vi "VNA-FMR_out-of-plane.vi"() -> ()   [LabVIEW 2015]
panel:
  out "Email Errors":string
  in  "File Comment":string
  in  "IF Bandwidth":string="10"
  in  "Stop":bool
  out "Status":string
  in  "Field Points":i32=1
  out "Current Set Point":dbl
  out "Current Output":dbl
  in  "Global Finished Email":bool
  in  "Save Directory":path=path "C:/Users/probe_station/Desktop/VNA-FMR_Data"
  in  "Scan Email":bool
  in  "Send File":bool
  out "Frequency":string
  out "Sweep Number":dbl
  out "Average IMAG":cluster{dbl[], dbl[]}(graph)
  out "Average REAL":cluster{dbl[], dbl[]}(graph)
  in  "Field Sweeps":i32=5
  out "Sweep IMAG":cluster{dbl[], dbl[]}(graph)
  out "Sweep REAL":cluster{dbl[], dbl[]}(graph)
  out "VNA IMAG":dbl
  out "Field (Oe)":dbl
  out "VNA REAL":dbl
  in  "FW Bell?":bool
  in  "Response Cal":bool=TRUE
  in  "Port Power Level":string="0"
  in  "Marker Sweep/Time Point":string="3ms"
  in  "VNA CW Sweep Time":string="min"
  in  "VNA number of Points":string="2"
  in  "Power Supply Address":string="1"
  in  "Current Start (A)":dbl
  in  "Current Stop (A)":dbl=70.0
  in  "VNA Address":string="15"
  in  "GaussMeter Address":string="12"
  in  "Start (GHz)":dbl=8.0
  in  "Stop (GHz)":dbl=9.0
  in  "Frequency Points":i32=2
  in  "Recipient's Email Address Address":string
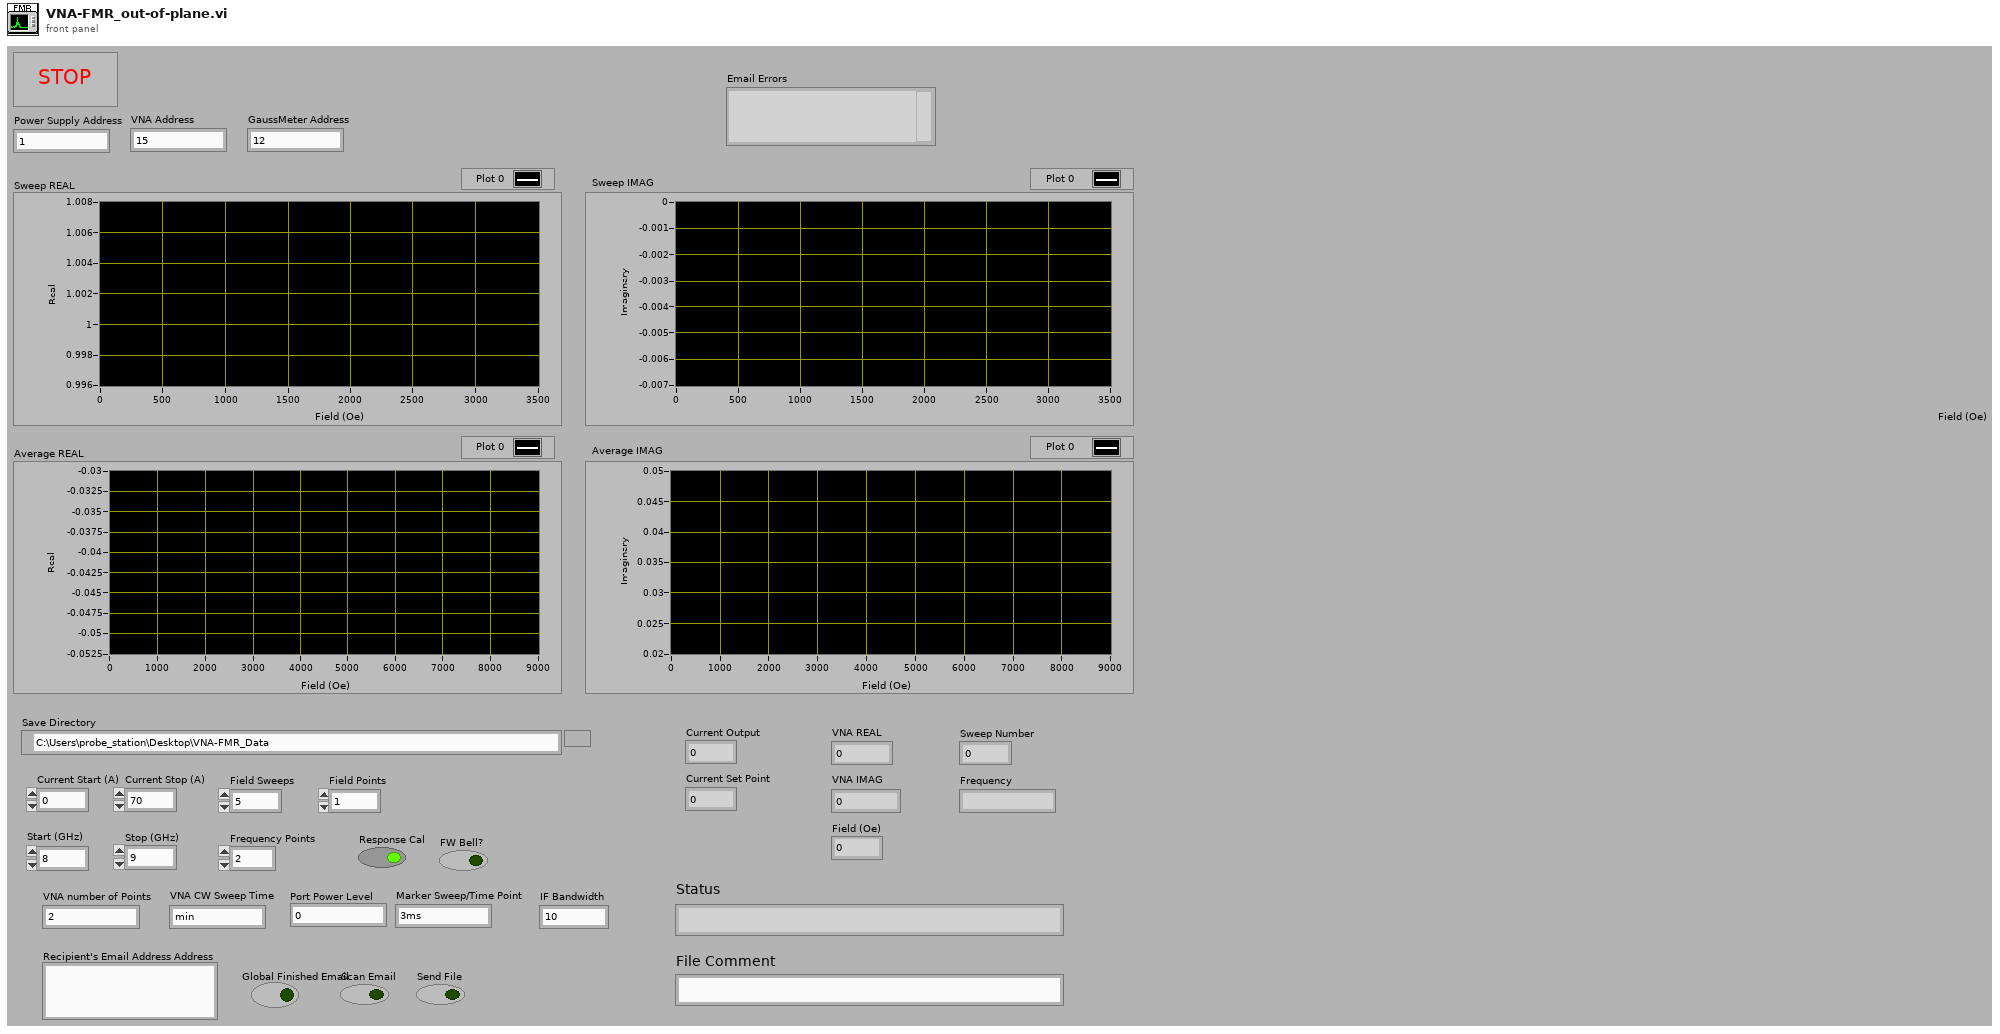
[diagram p1: front panel]
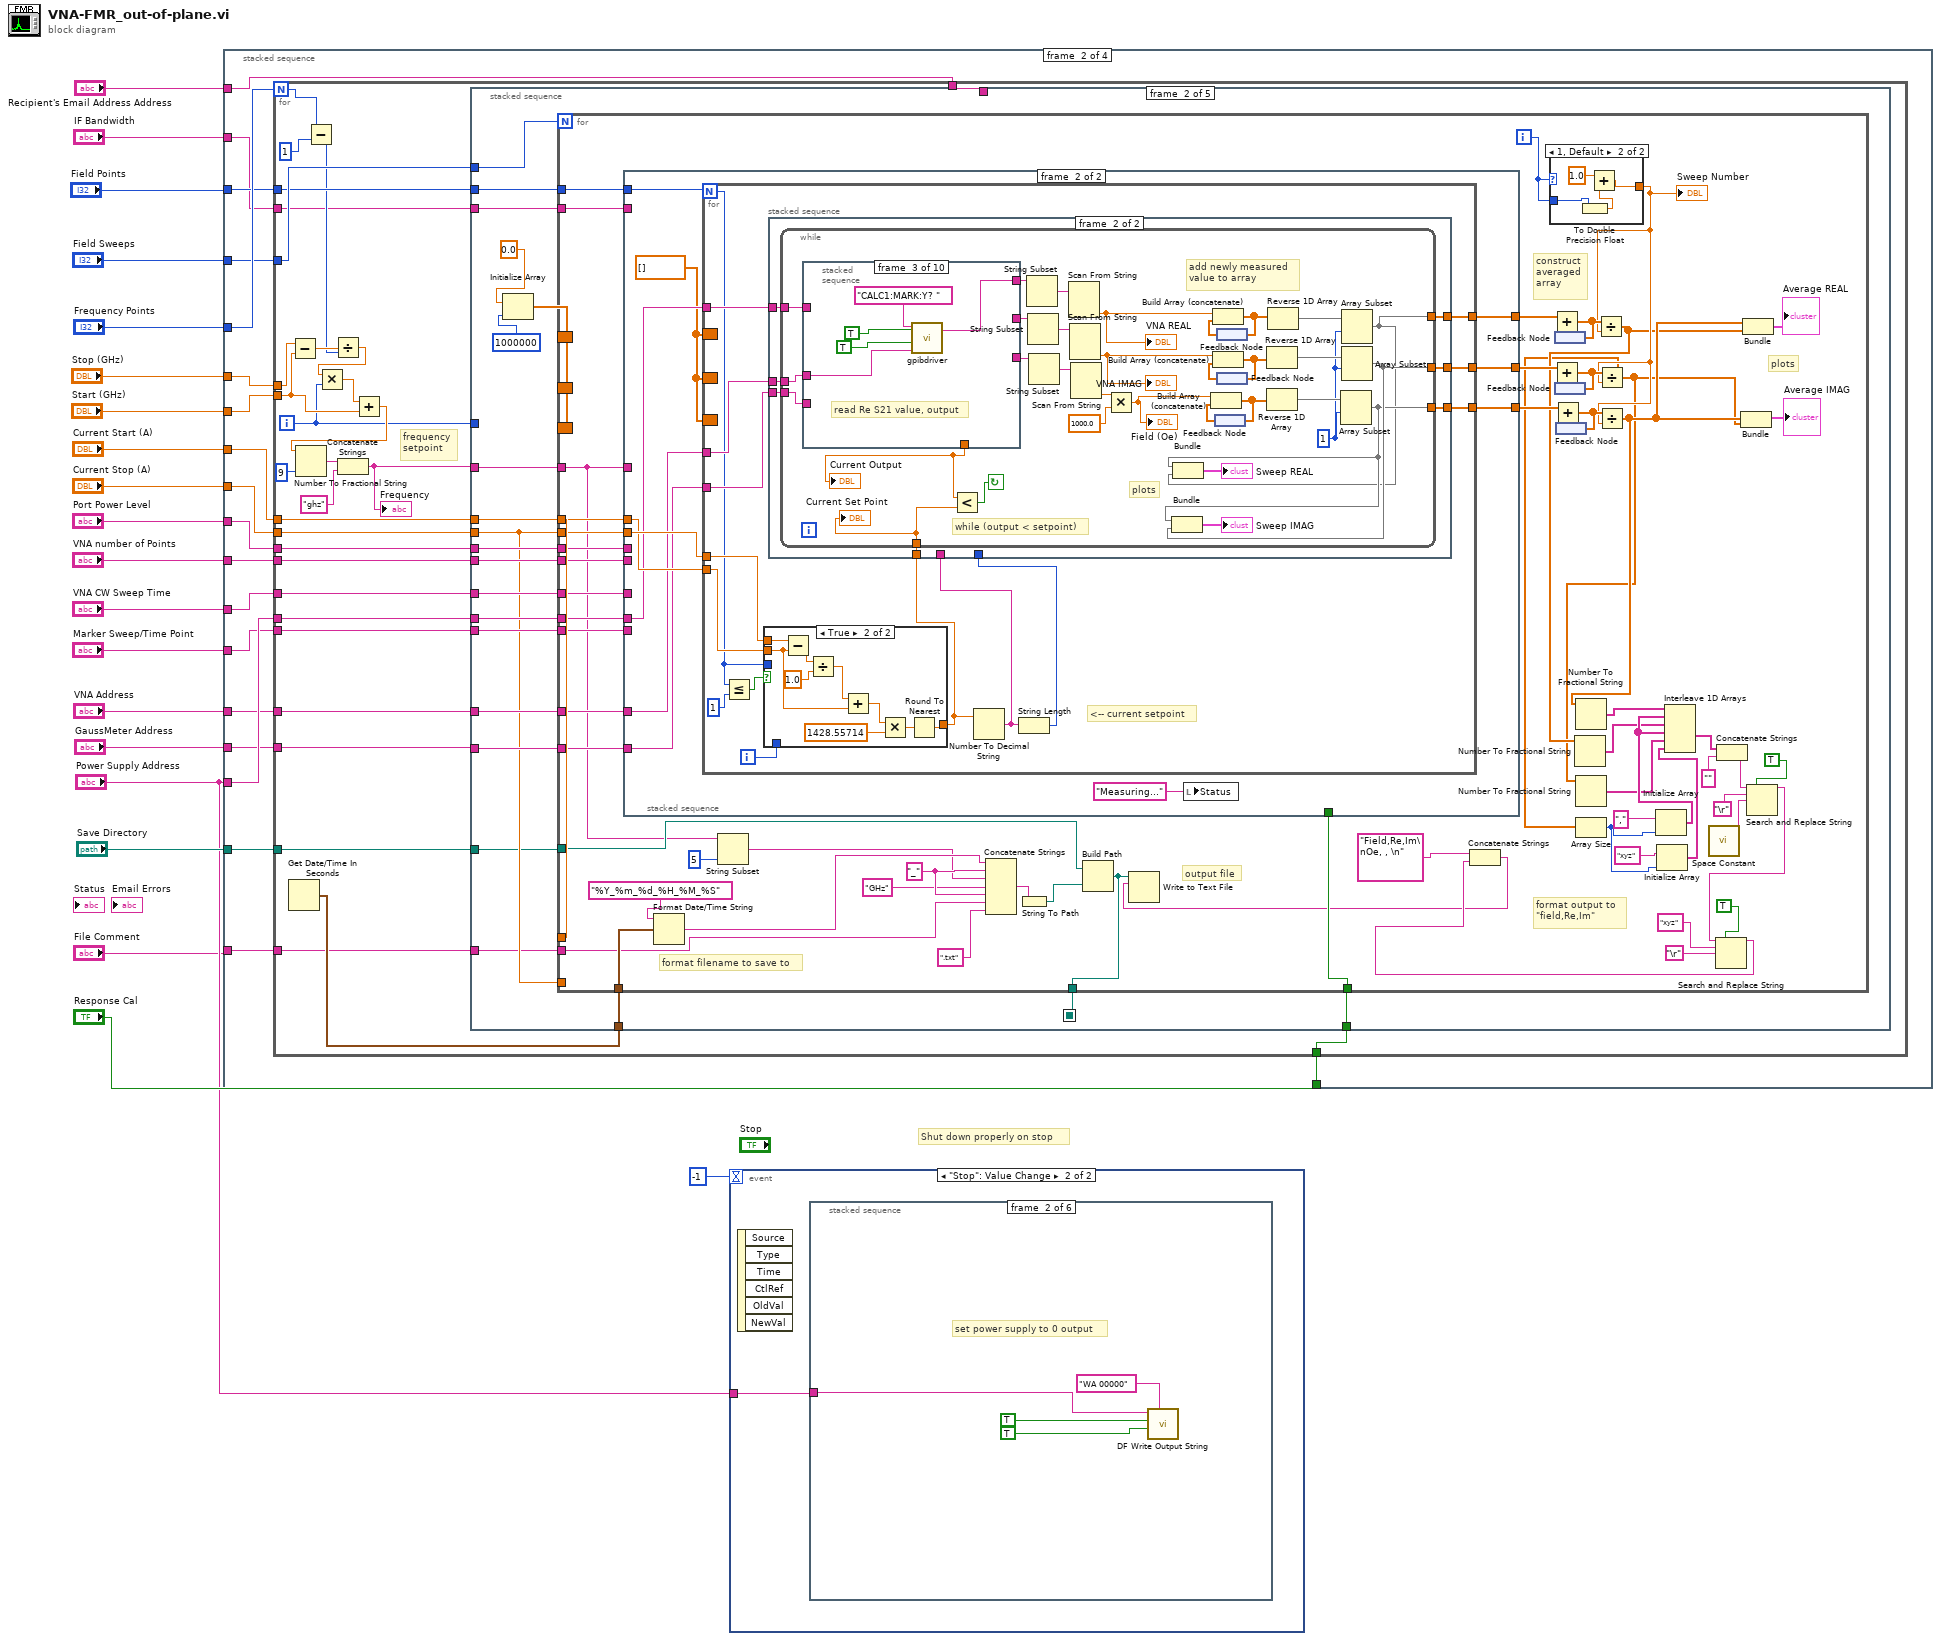
[diagram p0: block diagram]
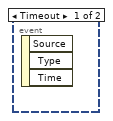
[diagram p2: hidden frame]
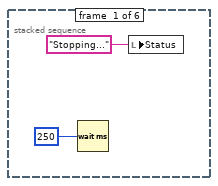
[diagram p3: hidden frame]
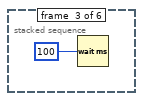
[diagram p4: hidden frame]
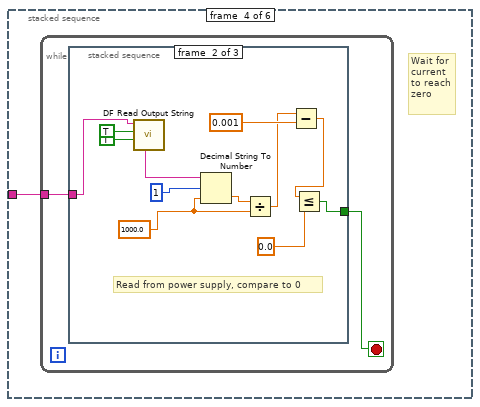
[diagram p5: hidden frame]
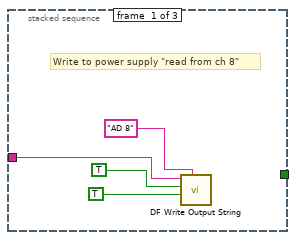
[diagram p6: hidden frame]
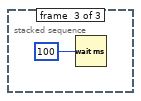
[diagram p7: hidden frame]
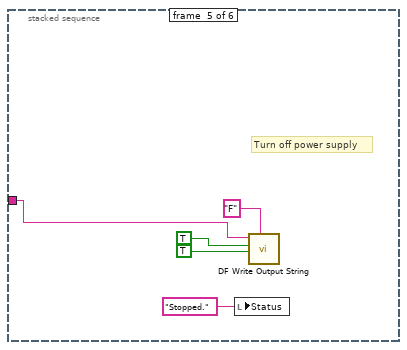
[diagram p8: hidden frame]
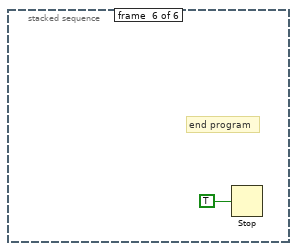
[diagram p9: hidden frame]
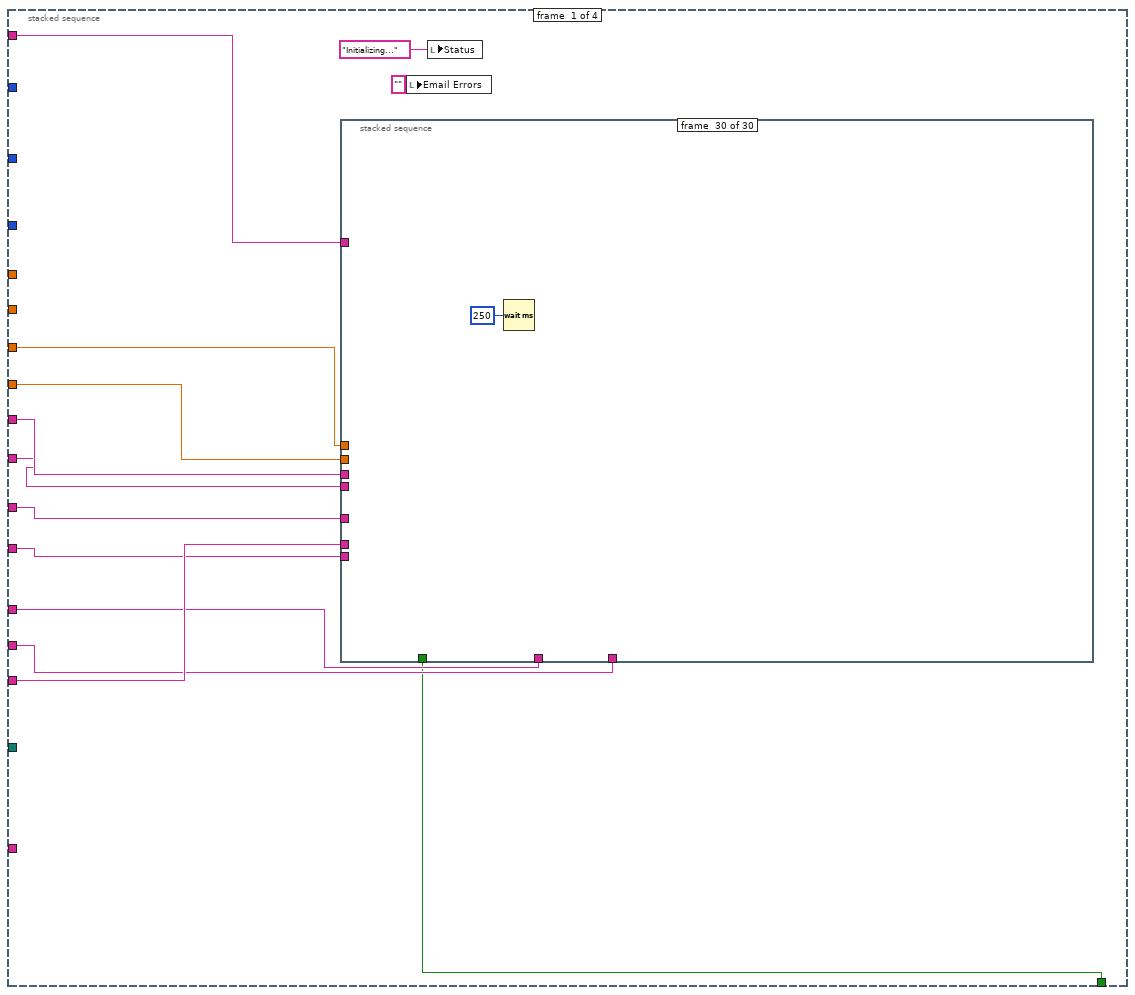
[diagram p10: hidden frame]
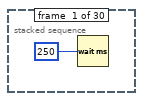
[diagram p11: hidden frame]
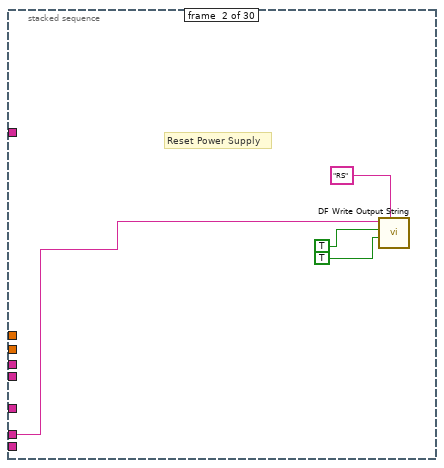
[diagram p12: hidden frame]
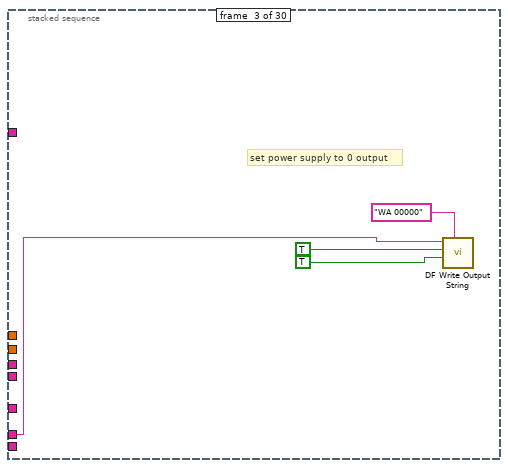
[diagram p13: hidden frame]
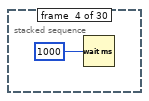
[diagram p14: hidden frame]
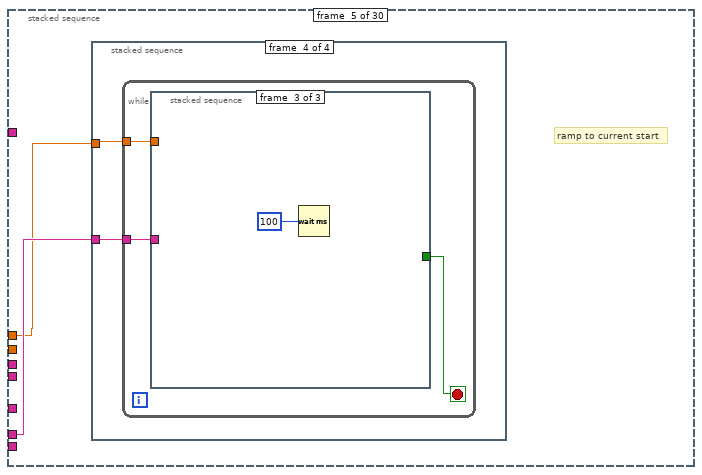
[diagram p15: hidden frame]
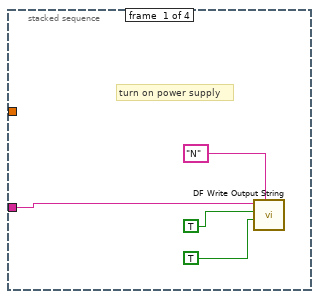
[diagram p16: hidden frame]
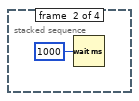
[diagram p17: hidden frame]
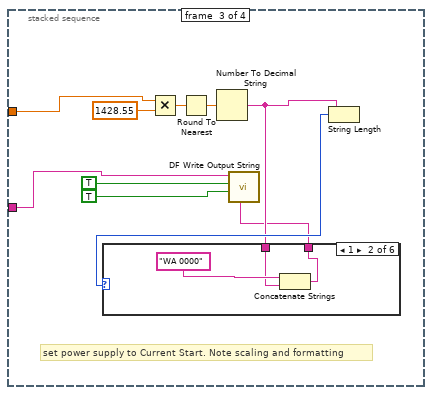
[diagram p18: hidden frame]
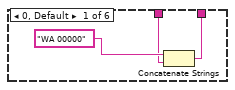
[diagram p19: hidden frame]
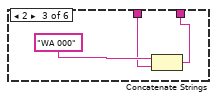
[diagram p20: hidden frame]
diagram:
  # "Shut down properly on stop"
  n1 = stacked-sequence {
    tunnel: "Recipient's Email Address Address" -> [_ w243 w824 _]
    tunnel: "Frequency Points" -> [_ w258 _ _]
    tunnel: "Stop (GHz)" -> [_ w257 _ _]
    tunnel: "Start (GHz)" -> [_ w256 _ _]
    tunnel: "Current Start (A)" -> [w33 w254 _ _]
    tunnel: "Current Stop (A)" -> [w32 w253 _ _]
    tunnel: "Port Power Level" -> [w31 w250 _ _]
    tunnel: "VNA number of Points" -> [w30 w251 _ _]
    tunnel: "VNA CW Sweep Time" -> [w29 w249 _ _]
    tunnel: "Marker Sweep/Time Point" -> [w27 w247 _ _]
    tunnel: "VNA Address" -> [w26 w252 _ _]
    tunnel: "Power Supply Address" -> [w28 w255 w823 _]
    tunnel: "GaussMeter Address" -> [w25 w246 _ _]
    tunnel: "Response Cal" -> [w24 w248 _ _]
    tunnel: "Field Points" -> [_ w245 _ _]
    tunnel: "Field Sweeps" -> [_ w244 _ _]
    tunnel: "Save Directory" -> [_ w242 _ _]
    tunnel: "IF Bandwidth" -> [w22 w241 _ _]
    tunnel: "File Comment" -> [_ w240 w821 _]
    frame #0 {
      n2 = stacked-sequence {
        tunnel: w28 -> [_ w38 w39 _ w45 _ _ _ _ _ _ _ _ _ _ _ _ _ _ _ _ _ _ _ _ _ _ _ _ _]
        tunnel: w33 -> [_ _ _ _ w44 _ _ _ _ _ _ _ _ _ _ _ _ _ _ _ _ _ _ _ _ _ _ _ _ _]
        tunnel: w32 -> [_ _ _ _ _ _ _ _ _ _ _ _ _ _ _ _ _ _ _ _ _ _ _ _ _ _ _ _ _ _]
        tunnel: w26 -> [_ _ _ _ _ w101 w105 w109 w115 w121 w127 w133 w137 w141 w145 w150 w156 w170 w174 w180 w184 w188 w193 w199 w213 w217 w221 w228 _ _]
        tunnel: w30 -> [_ _ _ _ _ _ _ w110 _ _ _ _ _ _ _ _ _ _ _ _ _ _ _ _ _ _ _ _ _ _]
        tunnel: w31 -> [_ _ _ _ _ _ _ _ w116 w122 _ _ _ _ _ _ _ _ _ _ _ _ _ _ _ _ _ _ _ _]
        tunnel: w29 -> [_ _ _ _ _ _ _ _ _ _ w128 _ _ _ _ _ _ _ _ _ _ _ _ _ _ _ _ _ _ _]
        tunnel: w24 -> [_ _ _ _ _ _ _ _ _ _ _ _ _ _ _ _ w155 _ _ _ _ _ _ w198 _ _ _ _ _ _]
        tunnel: w27 -> [_ _ _ _ _ _ _ _ _ _ _ _ _ _ _ _ _ _ w175 _ _ _ _ _ _ _ w222 _ _ _]
        tunnel: w25 -> [_ _ _ _ _ _ _ _ _ _ _ _ _ _ _ _ _ _ _ _ _ _ _ _ _ _ _ w227 w235 _]
        tunnel: w22 -> [_ _ _ _ _ _ _ _ _ _ _ _ _ _ _ w149 _ _ _ _ _ _ w192 _ _ _ _ _ _ _]
        frame #0 {
          n3 = Wait (ms)(milliseconds to wait=u32 250) -> ()  [unwired: 1 out]
        }
        frame #1 {
          # "Reset Power Supply"
          n4 = call "DF Write Output String"("Write String"="RS", "Communications Mode"=TRUE, "Communications On/Off"=TRUE, "GPIB Address"=w38) -> ()  [unwired: 5 in]
        }
        frame #2 {
          # "set power supply to 0 output"
          n5 = call "DF Write Output String"("Write String"="WA 00000", "Communications Mode"=TRUE, "Communications On/Off"=TRUE, "GPIB Address"=w39) -> ()  [unwired: 5 in]
        }
        frame #3 {
          n6 = Wait (ms)(milliseconds to wait=u32 1000) -> ()  [unwired: 1 out]
        }
        frame #4 {
          # "ramp to current start"
          n7 = stacked-sequence {
            tunnel: w45 -> [w46 _ w52 w80]
            tunnel: w44 -> [_ _ w51 w79]
            frame #0 {
              # "turn on power supply"
              n8 = call "DF Write Output String"("Write String"="N", "Communications Mode"=TRUE, "Communications On/Off"=TRUE, "GPIB Address"=w46) -> ()  [unwired: 5 in]
            }
            frame #1 {
              n9 = Wait (ms)(milliseconds to wait=u32 1000) -> ()  [unwired: 1 out]
            }
            frame #2 {
              # "set power supply to Current Start. Note scaling and formatting"
              n10 = Multiply(x=w51, y=1428.55) -> (x*y=w54:dbl)
              n11 = Round To Nearest(number=w54) -> (nearest integer value=w53:dbl)
              n12 = Number To Decimal String(number=w53) -> (decimal integer string=w56:string)  [unwired: 1 in]
              n13 = String Length(string=w56) -> (length=w57:i32)
              n14 = case shown="1" w57 {
                tunnel: w56 -> [w62 w65 w68 w71 w74 w77]
                tunnel: [w61 w64 w67 w70 w73 w76] -> w55
                frame 0, Default {
                  n15 = Concatenate Strings("WA 00000" ("string"), w62) -> (w61:string)
                }
                frame 1 {
                  n16 = Concatenate Strings("WA 0000" ("string"), w65) -> (w64:string)
                }
                frame 2 {
                  n17 = Concatenate Strings("WA 000" ("string"), w68) -> (w67:string)
                }
                frame 3 {
                  n18 = Concatenate Strings("WA 00" ("string"), w71) -> (w70:string)
                }
                frame 4 {
                  n19 = Concatenate Strings("WA 0" ("string"), w74) -> (w73:string)
                }
                frame 5 {
                  n20 = Concatenate Strings("WA " ("string"), w77) -> (w76:string)
                }
              }
              n21 = call "DF Write Output String"("Write String"=w55, "Communications Mode"=TRUE, "Communications On/Off"=TRUE, "GPIB Address"=w52) -> ()  [unwired: 5 in]
            }
            frame #3 {
              n22 = while {
                tunnel: w80 -> [w82]
                tunnel: w79 -> [w81]
                stop <- w83 stop-if-true
                n23 = stacked-sequence {
                  tunnel: [_ w93 _] -> w83
                  tunnel: w82 -> [w84 w89 _]
                  tunnel: w81 -> [_ w88 _]
                  frame #0 {
                    # "Write to power supply \"read from ch 8\""
                    n24 = call "DF Write Output String"("Write String"="AD 8", "Communications Mode"=TRUE, "Communications On/Off"=TRUE, "GPIB Address"=w84) -> ()  [unwired: 5 in]
                  }
                  frame #1 {
                    w96 = 1000.0 ("y")
                    # "Read from power supply, compare to\nsetpoint"
                    n25 = call "DF Read Output String"("Communications Mode"=TRUE, "Readback On/Off"=TRUE, "GPIB Address"=w89) -> ("Read String"=w97:string)  [unwired: 4 in, 1 out]
                    n26 = Decimal String To Number(string=w97, offset=1, default (0L)=w96) -> (number=w95:dbl)  [unwired: 1 out]
                    n27 = Divide(x=w95, y=w96) -> (x/y=w91:dbl)
                    n28 = Add(x=w91, y=0.001) -> (x+y=w90:dbl)
                    n29 = Greater Or Equal?(x=w90, y=w88) -> (x >= y?=w93:bool)
                  }
                  frame #2 {
                    n30 = Wait (ms)(milliseconds to wait=u32 100) -> ()  [unwired: 1 out]
                  }
                }
              }
            }
          }
        }
        frame #5 {
          # "send to VNA \"delete all measurements\""
          n31 = call "gpibdriver.vi"("Characters to Write"="CALC:PAR:DEL:ALL", "Read"=FALSE, "Write"=TRUE ("Write 3"), "GPIB\nAddress"=w101) -> ()  [unwired: 2 in, 1 out]
        }
        frame #6 {
          # "send to VNA \"set sweep type to CW\""
          n32 = call "gpibdriver.vi"("Characters to Write"="SENS1:SWE:TYPE CW", "Read"=FALSE, "Write"=TRUE ("Write 3"), "GPIB\nAddress"=w105) -> ()  [unwired: 2 in, 1 out]
        }
        frame #7 {
          # "Send to VNA \"set # of sweep points\"\naccepts number or min/max"
          n33 = Concatenate Strings("SENS:SWE:POIN " ("Characters to Write"), w110) -> (w111:string)
          n34 = call "gpibdriver.vi"("Characters to Write"=w111, "Read"=FALSE, "Write"=TRUE, "GPIB\nAddress"=w109) -> ()  [unwired: 2 in, 1 out]
        }
        frame #8 {
          # "send to VNA \"set port 1 power output\nto Port Power Level\" in dBm"
          n35 = Concatenate Strings("SOUR:POW1 " ("Characters to Write"), w116) -> (w117:string)
          n36 = call "gpibdriver.vi"("Characters to Write"=w117, "Read"=FALSE, "Write"=TRUE ("Write 3"), "GPIB\nAddress"=w115) -> ()  [unwired: 2 in, 1 out]
        }
        frame #9 {
          # "send to VNA \"set port 2 power output\nto Port Power Level\" in dBm"
          n37 = Concatenate Strings("SOUR:POW2 " ("Characters to Write"), w122) -> (w123:string)
          n38 = call "gpibdriver.vi"("Characters to Write"=w123, "Read"=FALSE, "Write"=TRUE ("Write 3"), "GPIB\nAddress"=w121) -> ()  [unwired: 2 in, 1 out]
        }
        frame #10 {
          # "set sweep time"
          n39 = Concatenate Strings("SENS:SWE:TIME " ("Characters to Write"), w128) -> (w129:string)
          n40 = call "gpibdriver.vi"("Characters to Write"=w129, "Read"=FALSE, "Write"=TRUE ("Write 3"), "GPIB\nAddress"=w127) -> ()  [unwired: 2 in, 1 out]
        }
        frame #11 {
          # "create new VNA measurement of S21"
          n41 = call "gpibdriver.vi"("Characters to Write"="CALC1:PAR:DEF \"CH1_S21_RE\", S21", "Read"=FALSE, "Write"=TRUE ("Write 3"), "GPIB\nAddress"=w133) -> ()  [unwired: 2 in, 1 out]
        }
        frame #12 {
          # "Display real S21 measurement on VNA"
          n42 = call "gpibdriver.vi"("Characters to Write"="DISP:WIND1:TRAC1:FEED \"CH1_S21_RE\"", "Read"=FALSE, "Write"=TRUE ("Write 3"), "GPIB\nAddress"=w137) -> ()  [unwired: 2 in, 1 out]
        }
        frame #13 {
          # "sets S21 measurement on VNA"
          n43 = call "gpibdriver.vi"("Characters to Write"="CALC1:PAR:SEL \"CH1_S21_RE\"", "Read"=FALSE, "Write"=TRUE ("Write 3"), "GPIB\nAddress"=w141) -> ()  [unwired: 2 in, 1 out]
        }
        frame #14 {
          # "display Real part of selected measurement (S21)"
          n44 = call "gpibdriver.vi"("Characters to Write"="CALC1:FORM REAL", "Read"=FALSE, "Write"=TRUE ("Write 3"), "GPIB\nAddress"=w145) -> ()  [unwired: 2 in, 1 out]
        }
        frame #15 {
          # "Set IF Bandwidth"
          n45 = Concatenate Strings("sense1:bandwidth " ("Characters to Write"), w149) -> (w151:string)
          n46 = call "gpibdriver.vi"("Characters to Write"=w151, "Read"=FALSE, "Write"=TRUE, "GPIB\nAddress"=w150) -> ()  [unwired: 2 in, 1 out]
        }
        frame #16 {
          # "Response Cal?"
          n47 = case shown="True" w155 {
            tunnel: w156 -> [_ w157]
            frame False {
            }
            frame True {
              n48 = stacked-sequence {
                tunnel: w157 -> [w158 w162 w166]
                frame #0 {
                  # "set ch 1 calibratoin to Response Thru"
                  n49 = call "gpibdriver.vi"("Characters to Write"="SENS:CORR:COLL:METH TRAN1", "Read"=FALSE, "Write"=TRUE, "GPIB\nAddress"=w158) -> ()  [unwired: 2 in, 1 out]
                }
                frame #1 {
                  # "measure the calibration standard\n(not 100% sure on this one)"
                  n50 = call "gpibdriver.vi"("Characters to Write"="SENS:CORR:COLL STAN4", "Read"=FALSE, "Write"=TRUE, "GPIB\nAddress"=w162) -> ()  [unwired: 2 in, 1 out]
                }
                frame #2 {
                  # "save calibration"
                  n51 = call "gpibdriver.vi"("Characters to Write"="SENS:CORR:COLL:SAVE", "Read"=FALSE, "Write"=TRUE, "GPIB\nAddress"=w166) -> ()  [unwired: 2 in, 1 out]
                }
              }
            }
          }
        }
        frame #17 {
          # "turns marker on ch 1\nnot 100% sure"
          n52 = call "gpibdriver.vi"("Characters to Write"="CALC1:MARK ON", "Read"=FALSE, "Write"=TRUE ("Write 3"), "GPIB\nAddress"=w170) -> ()  [unwired: 2 in, 1 out]
        }
        frame #18 {
          # "set ch1 marker to Marker Sweep/Time point"
          n53 = Concatenate Strings("CALC1:MARK:X " ("Characters to Write"), w175) -> (w176:string)
          n54 = call "gpibdriver.vi"("Characters to Write"=w176, "Read"=FALSE, "Write"=TRUE ("Write 3"), "GPIB\nAddress"=w174) -> ()  [unwired: 2 in, 1 out]
        }
        frame #19 {
          # "create new S21 measurement"
          n55 = call "gpibdriver.vi"("Characters to Write"="CALC1:PAR:DEF \"CH1_S21_IM\", S21", "Read"=FALSE, "Write"=TRUE ("Write 3"), "GPIB\nAddress"=w180) -> ()  [unwired: 2 in, 1 out]
        }
        frame #20 {
          # "display imaginary S21 measurement\non VNA"
          n56 = call "gpibdriver.vi"("Characters to Write"="DISP:WIND1:TRAC2:FEED \"CH1_S21_IM\"", "Read"=FALSE, "Write"=TRUE ("Write 3"), "GPIB\nAddress"=w184) -> ()  [unwired: 2 in, 1 out]
        }
        frame #21 {
          # "select Im S21 measurement"
          n57 = call "gpibdriver.vi"("Characters to Write"="CALC1:PAR:SEL \"CH1_S21_IM\"", "Read"=FALSE, "Write"=TRUE ("Write 3"), "GPIB\nAddress"=w188) -> ()  [unwired: 2 in, 1 out]
        }
        frame #22 {
          # "Set IF Bandwidth"
          n58 = Concatenate Strings("sense1:bandwidth " ("Characters to Write"), w192) -> (w194:string)
          n59 = call "gpibdriver.vi"("Characters to Write"=w194, "Read"=FALSE, "Write"=TRUE, "GPIB\nAddress"=w193) -> ()  [unwired: 2 in, 1 out]
        }
        frame #23 {
          # "response cal?"
          n60 = case shown="True" w198 {
            tunnel: w199 -> [_ w200]
            frame False {
            }
            frame True {
              n61 = stacked-sequence {
                tunnel: w200 -> [w201 w205 w209]
                frame #0 {
                  # "set calibratoin to response thru"
                  n62 = call "gpibdriver.vi"("Characters to Write"="SENS:CORR:COLL:METH TRAN1", "Read"=FALSE, "Write"=TRUE, "GPIB\nAddress"=w201) -> ()  [unwired: 2 in, 1 out]
                }
                frame #1 {
                  # "measure calibration?"
                  n63 = call "gpibdriver.vi"("Characters to Write"="SENS:CORR:COLL STAN4", "Read"=FALSE, "Write"=TRUE, "GPIB\nAddress"=w205) -> ()  [unwired: 2 in, 1 out]
                }
                frame #2 {
                  # "save calibration"
                  n64 = call "gpibdriver.vi"("Characters to Write"="SENS:CORR:COLL:SAVE", "Read"=FALSE, "Write"=TRUE, "GPIB\nAddress"=w209) -> ()  [unwired: 2 in, 1 out]
                }
              }
            }
          }
        }
        frame #24 {
          n65 = call "gpibdriver.vi"("Characters to Write"="CALC1:FORM IMAG", "Read"=FALSE, "Write"=TRUE ("Write 3"), "GPIB\nAddress"=w213) -> ()  [unwired: 2 in, 1 out]
        }
        frame #25 {
          n66 = call "gpibdriver.vi"("Characters to Write"="CALC1:MARK ON", "Read"=FALSE, "Write"=TRUE ("Write 3"), "GPIB\nAddress"=w217) -> ()  [unwired: 2 in, 1 out]
        }
        frame #26 {
          n67 = Concatenate Strings("CALC1:MARK:X " ("Characters to Write"), w222) -> (w223:string)
          n68 = call "gpibdriver.vi"("Characters to Write"=w223, "Read"=FALSE, "Write"=TRUE ("Write 3"), "GPIB\nAddress"=w221) -> ()  [unwired: 2 in, 1 out]
        }
        frame #27 {
          # "set fast data mode on gauss meter\nshould this be outside this structure/\nhigher level?"
          # "set manual sweep on VNA"
          n69 = call "gpibdriver.vi"("Characters to Write"="INIT:CONT OFF", "Read"=FALSE, "Write"=TRUE, "GPIB\nAddress"=w228) -> ()  [unwired: 2 in, 1 out]
          n70 = call "gpibdriver.vi"("Characters to Write"="fast 1", "Read"=FALSE, "Write"=TRUE, "GPIB\nAddress"=w227) -> ()  [unwired: 2 in, 1 out]
        }
        frame #28 {
          # "set highest range on gauss meter"
          n71 = call "gpibdriver.vi"("Characters to Write"="range 0", "Read"=FALSE, "Write"=TRUE ("Write 3"), "GPIB\nAddress"=w235) -> ()  [unwired: 2 in, 1 out]
        }
        frame #29 {
          n72 = Wait (ms)(milliseconds to wait=u32 250) -> ()  [unwired: 1 out]
        }
      }
      n73 = local write "Email Errors"("" ("Errors")) -> ()
      n74 = local write "Status"("Initializing..." ("Status")) -> ()
    }
    frame #1 {
      n75 = for {
        N: w258 -> [w263]
        tunnel: w257 -> [w289]
        tunnel: w256 -> [w285]
        tunnel: w255 -> [w280]
        tunnel: w254 -> [w279]
        tunnel: w253 -> [w278]
        tunnel: w252 -> [w277]
        tunnel: w251 -> [w276]
        tunnel: w250 -> [w275]
        tunnel: w249 -> [w274]
        tunnel: w248 -> [w273]
        tunnel: w247 -> [w272]
        tunnel: w246 -> [w271]
        tunnel: w245 -> [w265]
        tunnel: w244 -> [w270]
        tunnel: w243 -> [w268]
        tunnel: w242 -> [w264]
        tunnel: w241 -> [w260]
        tunnel: w240 -> [w259]
        i -> [w267]
        # "frequency\nsetpoint"
        n76 = Get Date/Time In Seconds() -> (seconds since 1Jan1904=w266:timestamp)
        n77 = Subtract(x=w289, y=w285) -> (x-y=w288:dbl)
        n78 = Subtract(x=w263, y=1) -> (x-y=w261:i32)
        n79 = Divide(x=w288, y=w261) -> (x/y=w287:dbl)
        n80 = Multiply(x=w287, y=w267) -> (x*y=w286:dbl)
        n81 = Add(x=w286, y=w285) -> (x+y=w281:dbl)
        n82 = Number To Fractional String(number=w281, precision (6)=i16 9) -> (F-format string=w284:string)  [unwired: 2 in]
        n83 = Concatenate Strings(w284, "ghz" ("string")) -> (w269:string)
        "Frequency" <- w269
        n84 = stacked-sequence {
          seq-local: [_ w312 _ _ _] -> [_ _ _ _ w781]
          tunnel: w280 -> [w295 w330 w776 _ _]
          tunnel: w279 -> [w300 w315 _ _ _]
          tunnel: w278 -> [w299 w314 _ _ _]
          tunnel: w277 -> [w293 w329 _ _ _]
          tunnel: w276 -> [w297 w328 _ _ _]
          tunnel: w275 -> [w298 w327 _ _ _]
          tunnel: w269 -> [w301 w326 _ _ w784]
          tunnel: w274 -> [w296 w325 _ _ _]
          tunnel: w273 -> [w291 w324 _ _ _]
          tunnel: w272 -> [w294 w323 _ _ _]
          tunnel: w271 -> [w292 w322 _ _ _]
          tunnel: w265 -> [_ w321 _ _ _]
          tunnel: w270 -> [_ w320 _ _ _]
          tunnel: w268 -> [_ _ _ _ w783]
          tunnel: w267 -> [_ _ _ _ w782]
          tunnel: w266 -> [_ w316 _ _ _]
          tunnel: w264 -> [_ w313 _ _ _]
          tunnel: w260 -> [_ w311 _ _ _]
          tunnel: w259 -> [_ w310 _ _ w780]
          frame #0 {
            n85 = stacked-sequence {
              tunnel: w295 -> [_ _ _]
              tunnel: w300 -> [_ _ _]
              tunnel: w299 -> [_ _ _]
              tunnel: w293 -> [_ w303 _]
              tunnel: w297 -> [_ _ _]
              tunnel: w298 -> [_ _ _]
              tunnel: w301 -> [_ w304 _]
              tunnel: w296 -> [_ _ _]
              tunnel: w291 -> [_ _ _]
              tunnel: w294 -> [_ _ _]
              tunnel: w292 -> [_ _ _]
              frame #0 {
                n86 = Wait (ms)(milliseconds to wait=u32 250) -> ()  [unwired: 1 out]
              }
              frame #1 {
                # "set VNA frequency to calculated frequency"
                n87 = Concatenate Strings("SENS:FREQ:CW " ("Characters to Write"), w304) -> (w306:string)
                n88 = call "gpibdriver.vi"("Characters to Write"=w306, "Read"=FALSE, "Write"=TRUE ("Write 3"), "GPIB\nAddress"=w303) -> ()  [unwired: 2 in, 1 out]
              }
              frame #2 {
                n89 = Wait (ms)(milliseconds to wait=u32 250) -> ()  [unwired: 1 out]
              }
            }
            n90 = local write "Status"("Preparing for next frequency sweep..." ("Status")) -> ()
          }
          frame #1 {
            n91 = Initialize Array(0.0 ("element"), 1000000 ("dimension size")) -> (w317:dbl[])
            n92 = for {
              N: w320 -> [_]
              tunnel: w330 -> [w393]
              tunnel: w315 -> [w392]
              tunnel: w314 -> [w391]
              tunnel: w329 -> [w390]
              tunnel: w328 -> [w389]
              tunnel: w327 -> [w388]
              tunnel: w326 -> [w335]
              tunnel: w325 -> [w387]
              tunnel: w324 -> [w386]
              tunnel: w323 -> [w385]
              tunnel: w322 -> [w384]
              tunnel: w321 -> [w383]
              border: w317 -> [_]
              border: w317 -> [_]
              border: w317 -> [_]
              tunnel: w316 -> [w368]
              tunnel: w315 -> [_]
              tunnel: w314 -> [_]
              tunnel: w313 -> [w366]
              tunnel: [w343] -> w312
              tunnel: w311 -> [w332]
              tunnel: w310 -> [w331]
              i -> [w371]
              w338 = "_" ("string")
              # "output file"
              # "format filename to save to"
              # "format output to\n\"field,Re,Im\""
              # "construct\naveraged\narray"
              # "plots"
              n93 = stacked-sequence {
                tunnel: w393 -> [w405 w622]
                tunnel: w392 -> [w401 w623]
                tunnel: w391 -> [_ w624]
                tunnel: w390 -> [w407 w620]
                tunnel: w389 -> [w403 _]
                tunnel: w388 -> [w402 _]
                tunnel: w335 -> [w399 _]
                tunnel: w387 -> [w404 _]
                tunnel: w386 -> [w409 _]
                tunnel: w385 -> [w406 _]
                tunnel: w384 -> [w408 w621]
                tunnel: w383 -> [_ w615]
                tunnel: [_ w618] -> w379
                tunnel: [_ w617] -> w378
                tunnel: [_ w616] -> w377
                tunnel: w332 -> [w400 _]
                frame #0 {
                  n94 = stacked-sequence {
                    tunnel: w405 -> [_ w412 _ w418 _ _ _ _ _ _ _ _ _ _ _ _ _ _ _ _ _ _ _ _ _ _ _ _ _ _]
                    tunnel: w401 -> [_ _ _ w417 _ _ _ _ _ _ _ _ _ _ _ _ _ _ _ _ _ _ _ _ _ _ _ _ _ _]
                    tunnel: w407 -> [_ _ _ _ w469 w473 w477 w483 w489 w495 w501 w507 w511 w515 w519 w524 w530 w544 w548 w554 w558 w562 w567 w573 w587 w591 w595 w602 _ _]
                    tunnel: w403 -> [_ _ _ _ _ _ w478 _ _ _ _ _ _ _ _ _ _ _ _ _ _ _ _ _ _ _ _ _ _ _]
                    tunnel: w402 -> [_ _ _ _ _ _ _ w484 w490 _ _ _ _ _ _ _ _ _ _ _ _ _ _ _ _ _ _ _ _ _]
                    tunnel: w404 -> [_ _ _ _ _ _ _ _ _ _ w502 _ _ _ _ _ _ _ _ _ _ _ _ _ _ _ _ _ _ _]
                    tunnel: w409 -> [_ _ _ _ _ _ _ _ _ _ _ _ _ _ _ _ w529 _ _ _ _ _ _ w572 _ _ _ _ _ _]
                    tunnel: w406 -> [_ _ _ _ _ _ _ _ _ _ _ _ _ _ _ _ _ _ w549 _ _ _ _ _ _ _ w596 _ _ _]
                    tunnel: w408 -> [_ _ _ _ _ _ _ _ _ _ _ _ _ _ _ _ _ _ _ _ _ _ _ _ _ _ _ w601 w609 _]
                    tunnel: w400 -> [_ _ _ _ _ _ _ _ _ _ _ _ _ _ _ w523 _ _ _ _ _ _ w566 _ _ _ _ _ _ _]
                    tunnel: w399 -> [_ _ _ _ _ _ _ _ _ w496 _ _ _ _ _ _ _ _ _ _ _ _ _ _ _ _ _ _ _ _]
                    frame #0 {
                      n95 = Wait (ms)(milliseconds to wait=u32 250) -> ()  [unwired: 1 out]
                    }
                    frame #1 {
                      # "set power supply to 0 output"
                      n96 = call "DF Write Output String"("Write String"="WA 00000", "Communications Mode"=TRUE, "Communications On/Off"=TRUE, "GPIB Address"=w412) -> ()  [unwired: 5 in]
                    }
                    frame #2 {
                      n97 = Wait (ms)(milliseconds to wait=u32 1000) -> ()  [unwired: 1 out]
                    }
                    frame #3 {
                      # "ramp to current start"
                      n98 = stacked-sequence {
                        tunnel: w418 -> [w420 w448]
                        tunnel: w417 -> [w419 w447]
                        frame #0 {
                          # "set power supply to Current Start. Note scaling and formatting"
                          n99 = Multiply(x=w419, y=1428.55) -> (x*y=w422:dbl)
                          n100 = Round To Nearest(number=w422) -> (nearest integer value=w421:dbl)
                          n101 = Number To Decimal String(number=w421) -> (decimal integer string=w424:string)  [unwired: 1 in]
                          n102 = String Length(string=w424) -> (length=w425:i32)
                          n103 = case shown="5" w425 {
                            tunnel: w424 -> [w430 w433 w436 w439 w442 w445]
                            tunnel: [w429 w432 w435 w438 w441 w444] -> w423
                            frame 0, Default {
                              n104 = Concatenate Strings("WA 00000" ("string"), w430) -> (w429:string)
                            }
                            frame 1 {
                              n105 = Concatenate Strings("WA 0000" ("string"), w433) -> (w432:string)
                            }
                            frame 2 {
                              n106 = Concatenate Strings("WA 000" ("string"), w436) -> (w435:string)
                            }
                            frame 3 {
                              n107 = Concatenate Strings("WA 00" ("string"), w439) -> (w438:string)
                            }
                            frame 4 {
                              n108 = Concatenate Strings("WA 0" ("string"), w442) -> (w441:string)
                            }
                            frame 5 {
                              n109 = Concatenate Strings("WA " ("string"), w445) -> (w444:string)
                            }
                          }
                          n110 = call "DF Write Output String"("Write String"=w423, "Communications Mode"=TRUE, "Communications On/Off"=TRUE, "GPIB Address"=w420) -> ()  [unwired: 5 in]
                        }
                        frame #1 {
                          n111 = while {
                            tunnel: w448 -> [w450]
                            tunnel: w447 -> [w449]
                            stop <- w451 stop-if-true
                            n112 = stacked-sequence {
                              tunnel: [_ w461 _] -> w451
                              tunnel: w450 -> [w452 w457 _]
                              tunnel: w449 -> [_ w456 _]
                              frame #0 {
                                # "Write to power supply \"read from ch 8\""
                                n113 = call "DF Write Output String"("Write String"="AD 8", "Communications Mode"=TRUE, "Communications On/Off"=TRUE, "GPIB Address"=w452) -> ()  [unwired: 5 in]
                              }
                              frame #1 {
                                w464 = 1000.0 ("y")
                                # "Read from power supply, compare to\nsetpoint"
                                n114 = call "DF Read Output String"("Communications Mode"=TRUE, "Readback On/Off"=TRUE, "GPIB Address"=w457) -> ("Read String"=w465:string)  [unwired: 4 in, 1 out]
                                n115 = Decimal String To Number(string=w465, offset=1, default (0L)=w464) -> (number=w463:dbl)  [unwired: 1 out]
                                n116 = Divide(x=w463, y=w464) -> (x/y=w459:dbl)
                                n117 = Subtract(x=w459, y=0.001) -> (x-y=w458:dbl)
                                n118 = Less Or Equal?(x=w458, y=w456) -> (x <= y?=w461:bool)
                              }
                              frame #2 {
                                n119 = Wait (ms)(milliseconds to wait=u32 100) -> ()  [unwired: 1 out]
                              }
                            }
                          }
                        }
                      }
                    }
                    frame #4 {
                      # "send to VNA \"delete all measurements\""
                      n120 = call "gpibdriver.vi"("Characters to Write"="CALC:PAR:DEL:ALL", "Read"=FALSE, "Write"=TRUE ("Write 3"), "GPIB\nAddress"=w469) -> ()  [unwired: 2 in, 1 out]
                    }
                    frame #5 {
                      # "send to VNA \"set sweep type to CW\""
                      n121 = call "gpibdriver.vi"("Characters to Write"="SENS1:SWE:TYPE CW", "Read"=FALSE, "Write"=TRUE ("Write 3"), "GPIB\nAddress"=w473) -> ()  [unwired: 2 in, 1 out]
                    }
                    frame #6 {
                      # "Send to VNA \"set # of sweep points\"\naccepts number or min/max"
                      n122 = Concatenate Strings("SENS:SWE:POIN " ("Characters to Write"), w478) -> (w479:string)
                      n123 = call "gpibdriver.vi"("Characters to Write"=w479, "Read"=FALSE, "Write"=TRUE, "GPIB\nAddress"=w477) -> ()  [unwired: 2 in, 1 out]
                    }
                    frame #7 {
                      # "send to VNA \"set port 1 power output\nto Port Power Level\" in dBm"
                      n124 = Concatenate Strings("SOUR:POW1 " ("Characters to Write"), w484) -> (w485:string)
                      n125 = call "gpibdriver.vi"("Characters to Write"=w485, "Read"=FALSE, "Write"=TRUE ("Write 3"), "GPIB\nAddress"=w483) -> ()  [unwired: 2 in, 1 out]
                    }
                    frame #8 {
                      # "send to VNA \"set port 2 power output\nto Port Power Level\" in dBm"
                      n126 = Concatenate Strings("SOUR:POW2 " ("Characters to Write"), w490) -> (w491:string)
                      n127 = call "gpibdriver.vi"("Characters to Write"=w491, "Read"=FALSE, "Write"=TRUE ("Write 3"), "GPIB\nAddress"=w489) -> ()  [unwired: 2 in, 1 out]
                    }
                    frame #9 {
                      # "set frequency"
                      n128 = Concatenate Strings("SENS:FREQ:CW " ("Characters to Write"), w496) -> (w500:string)
                      n129 = call "gpibdriver.vi"("Characters to Write"=w500, "Read"=FALSE, "Write"=TRUE ("Write 3"), "GPIB\nAddress"=w495) -> ()  [unwired: 2 in, 1 out]
                    }
                    frame #10 {
                      # "set sweep time"
                      n130 = Concatenate Strings("SENS:SWE:TIME " ("Characters to Write"), w502) -> (w503:string)
                      n131 = call "gpibdriver.vi"("Characters to Write"=w503, "Read"=FALSE, "Write"=TRUE ("Write 3"), "GPIB\nAddress"=w501) -> ()  [unwired: 2 in, 1 out]
                    }
                    frame #11 {
                      # "create new VNA measurement of S21"
                      n132 = call "gpibdriver.vi"("Characters to Write"="CALC1:PAR:DEF \"CH1_S21_RE\", S21", "Read"=FALSE, "Write"=TRUE ("Write 3"), "GPIB\nAddress"=w507) -> ()  [unwired: 2 in, 1 out]
                    }
                    frame #12 {
                      # "Display real S21 measurement on VNA"
                      n133 = call "gpibdriver.vi"("Characters to Write"="DISP:WIND1:TRAC1:FEED \"CH1_S21_RE\"", "Read"=FALSE, "Write"=TRUE ("Write 3"), "GPIB\nAddress"=w511) -> ()  [unwired: 2 in, 1 out]
                    }
                    frame #13 {
                      # "sets S21 measurement on VNA"
                      n134 = call "gpibdriver.vi"("Characters to Write"="CALC1:PAR:SEL \"CH1_S21_RE\"", "Read"=FALSE, "Write"=TRUE ("Write 3"), "GPIB\nAddress"=w515) -> ()  [unwired: 2 in, 1 out]
                    }
                    frame #14 {
                      # "display Real part of selected measurement (S21)"
                      n135 = call "gpibdriver.vi"("Characters to Write"="CALC1:FORM REAL", "Read"=FALSE, "Write"=TRUE ("Write 3"), "GPIB\nAddress"=w519) -> ()  [unwired: 2 in, 1 out]
                    }
                    frame #15 {
                      # "Set IF Bandwidth"
                      n136 = Concatenate Strings("sense1:bandwidth " ("Characters to Write"), w523) -> (w525:string)
                      n137 = call "gpibdriver.vi"("Characters to Write"=w525, "Read"=FALSE, "Write"=TRUE, "GPIB\nAddress"=w524) -> ()  [unwired: 2 in, 1 out]
                    }
                    frame #16 {
                      # "Response Cal?"
                      n138 = case shown="True" w529 {
                        tunnel: w530 -> [_ w531]
                        frame False {
                        }
                        frame True {
                          n139 = stacked-sequence {
                            tunnel: w531 -> [w532 w536 w540]
                            frame #0 {
                              # "set ch 1 calibratoin to Response Thru"
                              n140 = call "gpibdriver.vi"("Characters to Write"="SENS:CORR:COLL:METH TRAN1", "Read"=FALSE, "Write"=TRUE, "GPIB\nAddress"=w532) -> ()  [unwired: 2 in, 1 out]
                            }
                            frame #1 {
                              # "measure the calibration standard\n(not 100% sure on this one)"
                              n141 = call "gpibdriver.vi"("Characters to Write"="SENS:CORR:COLL STAN4", "Read"=FALSE, "Write"=TRUE, "GPIB\nAddress"=w536) -> ()  [unwired: 2 in, 1 out]
                            }
                            frame #2 {
                              # "save calibration"
                              n142 = call "gpibdriver.vi"("Characters to Write"="SENS:CORR:COLL:SAVE", "Read"=FALSE, "Write"=TRUE, "GPIB\nAddress"=w540) -> ()  [unwired: 2 in, 1 out]
                            }
                          }
                        }
                      }
                    }
                    frame #17 {
                      # "turns marker on ch 1\nnot 100% sure"
                      n143 = call "gpibdriver.vi"("Characters to Write"="CALC1:MARK ON", "Read"=FALSE, "Write"=TRUE ("Write 3"), "GPIB\nAddress"=w544) -> ()  [unwired: 2 in, 1 out]
                    }
                    frame #18 {
                      # "set ch1 marker to Marker Sweep/Time point"
                      n144 = Concatenate Strings("CALC1:MARK:X " ("Characters to Write"), w549) -> (w550:string)
                      n145 = call "gpibdriver.vi"("Characters to Write"=w550, "Read"=FALSE, "Write"=TRUE ("Write 3"), "GPIB\nAddress"=w548) -> ()  [unwired: 2 in, 1 out]
                    }
                    frame #19 {
                      # "create new S21 measurement"
                      n146 = call "gpibdriver.vi"("Characters to Write"="CALC1:PAR:DEF \"CH1_S21_IM\", S21", "Read"=FALSE, "Write"=TRUE ("Write 3"), "GPIB\nAddress"=w554) -> ()  [unwired: 2 in, 1 out]
                    }
                    frame #20 {
                      # "display imaginary S21 measurement\non VNA"
                      n147 = call "gpibdriver.vi"("Characters to Write"="DISP:WIND1:TRAC2:FEED \"CH1_S21_IM\"", "Read"=FALSE, "Write"=TRUE ("Write 3"), "GPIB\nAddress"=w558) -> ()  [unwired: 2 in, 1 out]
                    }
                    frame #21 {
                      # "select Im S21 measurement"
                      n148 = call "gpibdriver.vi"("Characters to Write"="CALC1:PAR:SEL \"CH1_S21_IM\"", "Read"=FALSE, "Write"=TRUE ("Write 3"), "GPIB\nAddress"=w562) -> ()  [unwired: 2 in, 1 out]
                    }
                    frame #22 {
                      # "Set IF Bandwidth"
                      n149 = Concatenate Strings("sense1:bandwidth " ("Characters to Write"), w566) -> (w568:string)
                      n150 = call "gpibdriver.vi"("Characters to Write"=w568, "Read"=FALSE, "Write"=TRUE, "GPIB\nAddress"=w567) -> ()  [unwired: 2 in, 1 out]
                    }
                    frame #23 {
                      # "response cal?"
                      n151 = case shown="True" w572 {
                        tunnel: w573 -> [_ w574]
                        frame False {
                        }
                        frame True {
                          n152 = stacked-sequence {
                            tunnel: w574 -> [w575 w579 w583]
                            frame #0 {
                              # "set calibratoin to response thru"
                              n153 = call "gpibdriver.vi"("Characters to Write"="SENS:CORR:COLL:METH TRAN1", "Read"=FALSE, "Write"=TRUE, "GPIB\nAddress"=w575) -> ()  [unwired: 2 in, 1 out]
                            }
                            frame #1 {
                              # "measure calibration?"
                              n154 = call "gpibdriver.vi"("Characters to Write"="SENS:CORR:COLL STAN4", "Read"=FALSE, "Write"=TRUE, "GPIB\nAddress"=w579) -> ()  [unwired: 2 in, 1 out]
                            }
                            frame #2 {
                              # "save calibration"
                              n155 = call "gpibdriver.vi"("Characters to Write"="SENS:CORR:COLL:SAVE", "Read"=FALSE, "Write"=TRUE, "GPIB\nAddress"=w583) -> ()  [unwired: 2 in, 1 out]
                            }
                          }
                        }
                      }
                    }
                    frame #24 {
                      n156 = call "gpibdriver.vi"("Characters to Write"="CALC1:FORM IMAG", "Read"=FALSE, "Write"=TRUE ("Write 3"), "GPIB\nAddress"=w587) -> ()  [unwired: 2 in, 1 out]
                    }
                    frame #25 {
                      n157 = call "gpibdriver.vi"("Characters to Write"="CALC1:MARK ON", "Read"=FALSE, "Write"=TRUE ("Write 3"), "GPIB\nAddress"=w591) -> ()  [unwired: 2 in, 1 out]
                    }
                    frame #26 {
                      n158 = Concatenate Strings("CALC1:MARK:X " ("Characters to Write"), w596) -> (w597:string)
                      n159 = call "gpibdriver.vi"("Characters to Write"=w597, "Read"=FALSE, "Write"=TRUE ("Write 3"), "GPIB\nAddress"=w595) -> ()  [unwired: 2 in, 1 out]
                    }
                    frame #27 {
                      # "set fast data mode on gauss meter\nshould this be outside this structure/\nhigher level?"
                      # "set manual sweep on VNA"
                      n160 = call "gpibdriver.vi"("Characters to Write"="INIT:CONT OFF", "Read"=FALSE, "Write"=TRUE, "GPIB\nAddress"=w602) -> ()  [unwired: 2 in, 1 out]
                      n161 = call "gpibdriver.vi"("Characters to Write"="fast 1", "Read"=FALSE, "Write"=TRUE, "GPIB\nAddress"=w601) -> ()  [unwired: 2 in, 1 out]
                    }
                    frame #28 {
                      # "set highest range on gauss meter"
                      n162 = call "gpibdriver.vi"("Characters to Write"="range 0", "Read"=FALSE, "Write"=TRUE ("Write 3"), "GPIB\nAddress"=w609) -> ()  [unwired: 2 in, 1 out]
                    }
                    frame #29 {
                      n163 = Wait (ms)(milliseconds to wait=u32 1000) -> ()  [unwired: 1 out]
                    }
                  }
                  n164 = local write "Status"("Preparing for next field sweep..." ("Status")) -> ()
                }
                frame #1 {
                  w619 = dbl[] []
                  n165 = for {
                    N: w615 -> [w626]
                    tunnel: w624 -> [w629]
                    tunnel: w623 -> [w630]
                    tunnel: w622 -> [w639]
                    tunnel: w621 -> [w637]
                    tunnel: w620 -> [w636]
                    border: w619 -> [_]
                    border: w619 -> [_]
                    border: w619 -> [_]
                    tunnel: [w635] -> w618
                    tunnel: [w634] -> w617
                    tunnel: [w633] -> w616
                    i -> [w628]
                    # "<-- current setpoint"
                    n166 = Less Or Equal?(x=w626, y=1) -> (x <= y?=w631:bool)
                    n167 = case shown="True" w631 {
                      tunnel: w626 -> [w640 _]
                      tunnel: w630 -> [w644 w655]
                      tunnel: w629 -> [w643 w654]
                      tunnel: w628 -> [w642 _]
                      tunnel: [w641 w653] -> w627
                      frame False {
                        n168 = Subtract(x=w643, y=w644) -> (x-y=w649:dbl)
                        n169 = Divide(x=w649, y=w640) -> (x/y=w646:dbl)
                        n170 = Multiply(x=w646, y=w642) -> (x*y=w645:dbl)
                        n171 = Add(x=w645, y=w644) -> (x+y=w648:dbl)
                        n172 = Multiply(x=w648, y=1428.55714) -> (x*y=w647:dbl)
                        n173 = Round To Nearest(number=w647) -> (nearest integer value=w641:dbl)
                      }
                      frame True {
                        n174 = Subtract(x=w654, y=w655) -> (x-y=w658:dbl)
                        n175 = Divide(x=w658, y=1.0) -> (x/y=w652:dbl)
                        n176 = Add(x=w652, y=w655) -> (x+y=w657:dbl)
                        n177 = Multiply(x=w657, y=1428.55714) -> (x*y=w656:dbl)
                        n178 = Round To Nearest(number=w656) -> (nearest integer value=w653:dbl)
                      }
                    }
                    n179 = Number To Decimal String(number=w627) -> (decimal integer string=w632:string)  [unwired: 1 in]
                    n180 = String Length(string=w632) -> (length=w638:i32)
                    n181 = stacked-sequence {
                      tunnel: w639 -> [w663 w685]
                      tunnel: w638 -> [w662 _]
                      tunnel: w632 -> [w660 _]
                      tunnel: w637 -> [_ w690]
                      tunnel: w636 -> [_ w689]
                      tunnel: [_ w688] -> w635
                      tunnel: [_ w687] -> w634
                      tunnel: [_ w686] -> w633
                      tunnel: w627 -> [_ w684]
                      frame #0 {
                        # "set powersupply to current setpoint"
                        n182 = case shown="0, Default" w662 {
                          tunnel: [w667 w670 w673 w676 w679 w682] -> w661
                          tunnel: w660 -> [w666 w669 w672 w675 w678 w681]
                          frame 0, Default {
                            n183 = Concatenate Strings("WA 00000" ("string"), w666) -> (w667:string)
                          }
                          frame 1 {
                            n184 = Concatenate Strings("WA 0000" ("string"), w669) -> (w670:string)
                          }
                          frame 2 {
                            n185 = Concatenate Strings("WA 000" ("string"), w672) -> (w673:string)
                          }
                          frame 3 {
                            n186 = Concatenate Strings("WA 00" ("string"), w675) -> (w676:string)
                          }
                          frame 4 {
                            n187 = Concatenate Strings("WA 0" ("string"), w678) -> (w679:string)
                          }
                          frame 5 {
                            n188 = Concatenate Strings("WA " ("string"), w681) -> (w682:string)
                          }
                        }
                        n189 = call "DF Write Output String"("Write String"=w661, "Communications Mode"=TRUE, "Communications On/Off"=TRUE, "GPIB Address"=w663) -> ()  [unwired: 5 in]
                      }
                      frame #1 {
                        n190 = while {
                          tunnel: w690 -> [w722]
                          tunnel: w689 -> [w721]
                          tunnel: [w698] -> w688
                          tunnel: [w700] -> w687
                          tunnel: [w699] -> w686
                          tunnel: w685 -> [w697]
                          tunnel: w684 -> [w695]
                          stop <- w696 continue-if-true
                          w703 = 1 ("index")
                          # "add newly measured\nvalue to array"
                          # "while (output < setpoint)"
                          # "plots"
                          n191 = stacked-sequence {
                            tunnel: w722 -> [_ _ _ _ _ w747 _ _ _ _]
                            tunnel: w721 -> [w723 w727 w732 w736 w741 _ w756 _ _ _]
                            tunnel: [_ _ w731 _ _ _ _ _ _ _] -> w720
                            tunnel: [_ _ _ _ w740 _ _ _ _ _] -> w719
                            tunnel: [_ _ _ _ _ w746 _ _ _ _] -> w718
                            tunnel: w697 -> [_ _ _ _ _ _ _ w763 _ w772]
                            tunnel: [_ _ _ _ _ _ _ _ _ w766] -> w694
                            frame #0 {
                              # "send trigger to VNA"
                              n192 = call "gpibdriver.vi"("Characters to Write"="INIT", "Read"=FALSE, "Write"=TRUE ("Write 2"), "GPIB\nAddress"=w723) -> ()  [unwired: 2 in, 1 out]
                            }
                            frame #1 {
                              # "select Re S21 measurement"
                              n193 = call "gpibdriver.vi"("Characters to Write"="CALC1:PAR:SEL \"CH1_S21_RE\"", "Read"=FALSE, "Write"=TRUE ("Write 2"), "GPIB\nAddress"=w727) -> ()  [unwired: 2 in, 1 out]
                            }
                            frame #2 {
                              # "read Re S21 value, output"
                              n194 = call "gpibdriver.vi"("Characters to Write"="CALC1:MARK:Y? ", "Read"=TRUE, "Write"=TRUE ("Write 3"), "GPIB\nAddress"=w732) -> ("Characters Read"=w731:string)  [unwired: 2 in]
                            }
                            frame #3 {
                              # "select Im S21 measurement"
                              n195 = call "gpibdriver.vi"("Characters to Write"="CALC1:PAR:SEL \"CH1_S21_IM\"", "Read"=FALSE, "Write"=TRUE ("Write 3"), "GPIB\nAddress"=w736) -> ()  [unwired: 2 in, 1 out]
                            }
                            frame #4 {
                              # "read Im S21 value, output"
                              n196 = call "gpibdriver.vi"("Characters to Write"="CALC1:MARK:Y? ", "Read"=TRUE, "Write"=TRUE ("Write 3"), "GPIB\nAddress"=w741) -> ("Characters Read"=w740:string)  [unwired: 2 in]
                            }
                            frame #5 {
                              # "read field value, output"
                              n197 = case shown="False" "FW Bell?" {
                                tunnel: w747 -> [w749 _]
                                tunnel: [w748 w754] -> w746
                                frame False {
                                n198 = call "gpibdriver.vi"("Characters to Write"="field?", "Read"=TRUE, "Write"=TRUE ("Write 2"), "GPIB\nAddress"=w749) -> ("Characters Read"=w748:string)  [unwired: 2 in]
                                }
                                frame True {
                                n199 = call "read_gauss.vi"("Address of Gaussmeter"="10") -> ("Value (Gauss)"=w755:sgl)
                                n200 = Number To Fractional String(number=w755) -> (F-format string=w754:string)  [unwired: 3 in]
                                }
                              }
                            }
                            frame #6 {
                              # "operation complete?"
                              n201 = call "gpibdriver.vi"("Characters to Write"="*OPC?", "Read"=TRUE, "Write"=TRUE ("Write 2"), "GPIB\nAddress"=w756) -> ()  [unwired: 2 in, 1 out]
                            }
                            frame #7 {
                              # "read ch 8 from power supply"
                              n202 = call "DF Write Output String"("Write String"="AD 8", "Communications Mode"=TRUE, "Communications On/Off"=TRUE, "GPIB Address"=w763) -> ()  [unwired: 5 in]
                            }
                            frame #8 {
                              n203 = Wait (ms)(milliseconds to wait=u32 5) -> ()  [unwired: 1 out]
                            }
                            frame #9 {
                              # "find Current Output, output"
                              n204 = call "DF Read Output String"("Communications Mode"=TRUE, "Readback On/Off"=TRUE, "GPIB Address"=w772) -> ("Read String"=w769:string)  [unwired: 4 in, 1 out]
                              n205 = Decimal String To Number(string=w769, offset=1) -> (number=w767:i32)  [unwired: 1 in, 1 out]
                              n206 = Multiply(x=w767, y=1.43) -> (x*y=w766:dbl)
                            }
                          }
                          "Current Output" <- w694
                          n207 = Less?(x=w694, y=w695) -> (x < y?=w696:bool)
                          n208 = String Subset(string=w720) -> (substring=w716:string)  [unwired: 2 in]
                          n209 = String Subset(string=w719) -> (substring=w715:string)  [unwired: 2 in]
                          n210 = String Subset(string=w718) -> (substring=w717:string)  [unwired: 2 in]
                          n211 = Scan From String(input string=w716) -> (output 1=w710:dbl)  [unwired: 4 in, 3 out]
                          "VNA REAL" <- w710
                          n212 = Scan From String(input string=w715) -> (output 1=w711:dbl)  [unwired: 4 in, 3 out]
                          "VNA IMAG" <- w711
                          n213 = Scan From String(input string=w717) -> (output 1=w692:dbl)  [unwired: 4 in, 3 out]
                          n214 = Multiply(x=w692, y=1000.0) -> (x*y=w691:dbl)
                          "Field (Oe)" <- w691
                          n215 = feedback #1() -> (w714:dbl[])
                          n216 = Build Array (concatenate)(w691, w714) -> (w707:dbl[])
                          n217 = feedback-in #1(w707) -> ()
                          n218 = feedback #2() -> (w712:dbl[])
                          n219 = Build Array (concatenate)(w710, w712) -> (w708:dbl[])
                          n220 = feedback-in #2(w708) -> ()
                          n221 = feedback #3() -> (w713:dbl[])
                          n222 = Build Array (concatenate)(w711, w713) -> (w709:dbl[])
                          n223 = feedback-in #3(w709) -> ()
                          n224 = Reverse 1D Array(array=w709) -> (reversed array=w705:dbl[])
                          n225 = Reverse 1D Array(array=w707) -> (reversed array=w704:dbl[])
                          n226 = Reverse 1D Array(array=w708) -> (reversed array=w706:dbl[])
                          n227 = Array Subset(array=w704, index=w703) -> (w699:dbl[])  [unwired: 1 in]
                          n228 = Array Subset(array=w706, index=w703) -> (w698:dbl[])  [unwired: 1 in]
                          n229 = Bundle(w699, w698) -> (→"Sweep REAL":cluster{dbl[], dbl[]})  [unwired: 1 in]
                          n230 = Array Subset(array=w705, index=w703) -> (w700:dbl[])  [unwired: 1 in]
                          n231 = Bundle(w699, w700) -> (→"Sweep IMAG":cluster{dbl[], dbl[]})  [unwired: 1 in]
                          "Current Set Point" <- w695
                        }
                      }
                    }
                  }
                  n232 = local write "Status"("Measuring..." ("Status")) -> ()
                }
              }
              n233 = Format Date/Time String(time format string (%c)="%Y_%m_%d_%H_%M_%S", seconds (now)=w368) -> (date/time string=w342:string)  [unwired: 1 in]
              n234 = String Subset(string=w335, length (rest)=5 ("length (rest)")) -> (substring=w334:string)  [unwired: 1 in]
              n235 = Concatenate Strings(w342, w338, w334, "GHz" ("string"), w338, w331, ".txt" ("string")) -> (w367:string)
              n236 = String To Path(string=w367) -> (path=w365:path)
              n237 = Build Path(base path=w366, name or relative path=w365) -> (appended path=w343:path)
              n238 = case shown="1, Default" w371 {
                tunnel: [1.0 ("y") w395] -> w370
                tunnel: w371 -> [_ w398]
                frame 0 {
                }
                frame 1, Default {
                  n239 = To Double Precision Float(number=w398) -> (double precision float=w396:dbl)
                  n240 = Add(x=1.0, y=w396) -> (x+y=w395:dbl)
                }
              }
              "Sweep Number" <- w370
              n241 = feedback #4() -> (w382:dbl[])
              n242 = Add(x=w379, y=w382) -> (x+y=w376:dbl[])
              n243 = feedback-in #4(w376) -> ()
              n244 = feedback #5() -> (w381:dbl[])
              n245 = Add(x=w378, y=w381) -> (x+y=w375:dbl[])
              n246 = feedback-in #5(w375) -> ()
              n247 = feedback #6() -> (w380:dbl[])
              n248 = Add(x=w377, y=w380) -> (x+y=w374:dbl[])
              n249 = feedback-in #6(w374) -> ()
              n250 = Divide(x=w376, y=w370) -> (x/y=w363:dbl[])
              n251 = Number To Fractional String(number=w363) -> (F-format string=w346:string[])  [unwired: 3 in]
              n252 = Divide(x=w375, y=w370) -> (x/y=w362:dbl[])
              n253 = Number To Fractional String(number=w362) -> (F-format string=w345:string[])  [unwired: 3 in]
              n254 = Array Size(array=w362) -> (size(s)=w344:i32)
              n255 = Divide(x=w374, y=w370) -> (x/y=w364:dbl[])
              n256 = Number To Fractional String(number=w364) -> (F-format string=w347:string[])  [unwired: 3 in]
              n257 = Initialize Array(",", w344) -> (w349:string[])
              n258 = Initialize Array("xyz" ("element"), w344) -> (w350:string[])
              n259 = Interleave 1D Arrays(w347, w349, w346, w349, w345, w350) -> (w352:string[])
              n260 = call <vilib>:"Space Constant.vi"() -> ("String"=w361:string)
              n261 = Concatenate Strings(w352, "" ("string")) -> (w353:string)
              n262 = Bundle(w364, w362) -> (→"Average IMAG":cluster{dbl[], dbl[]})  [unwired: 1 in]
              n263 = Bundle(w364, w363) -> (→"Average REAL":cluster{dbl[], dbl[]})  [unwired: 1 in]
              n264 = Search and Replace String(replace all?=TRUE ("replace all? (F)"), input string=w353, search string="\r", replace string=w361) -> (result string=w355:string)  [unwired: 4 in, 3 out]
              n265 = Search and Replace String(replace all?=TRUE ("replace all? (F)"), input string=w355, search string="xyz", replace string="\r") -> (result string=w340:string)  [unwired: 4 in, 3 out]
              n266 = Concatenate Strings("Field,Re,Im\nOe, , \n" ("string"), w340) -> (w339:string)
              n267 = Write to Text File(file (use dialog)=w343, text=w339) -> ()  [unwired: 2 in, 3 out]
            }
          }
          frame #2 {
            # "turn off power supply"
            n268 = local write "Status"("Finishing frequency point..." ("Status")) -> ()
            n269 = call "DF Write Output String"("Write String"="WA 00000", "Communications Mode"=TRUE, "Communications On/Off"=TRUE, "GPIB Address"=w776) -> ()  [unwired: 5 in]
          }
          frame #3 {
            n270 = Wait (ms)(milliseconds to wait=u32 1000) -> ()  [unwired: 1 out]
          }
          frame #4 {
            n271 = case shown="True" "Scan Email" {
              tunnel: w784 -> [_ w801]
              tunnel: w783 -> [_ w800]
              tunnel: w782 -> [_ w799]
              tunnel: w781 -> [_ w798]
              tunnel: w780 -> [_ w797]
              tunnel: [_ w796] -> w779
              frame False {
              }
              frame True {
                n272 = case shown="True" "Send File" {
                  tunnel: w801 -> [w809 w819]
                  tunnel: w800 -> [w808 w816]
                  tunnel: w799 -> [_ _]
                  tunnel: w798 -> [_ w815]
                  tunnel: w797 -> [w804 w813]
                  tunnel: [w803 w811] -> w796
                  frame False {
                    n273 = Concatenate Strings("VNA-FMR System Message " ("Subject"), w804) -> (w805:string)
                    n274 = Concatenate Strings(w804, " Scan Finished @ " ("Body"), w809) -> (w807:string)
                    n275 = call "gmail 8.2.vi"("Subject"=w805, "Body"=w807, "Recipient's Email Address Address"=w808) -> ("error out"=w803:errorcluster)  [unwired: 8 in]
                  }
                  frame True {
                    n276 = Concatenate Strings(w813, " Scan Finished @ " ("Body"), w819) -> (w817:string)
                    n277 = Concatenate Strings("VNA-FMR System Message " ("Subject"), w813) -> (w812:string)
                    n278 = call "gmail 8.2.vi"("Attachment - Optional"=w815, "Subject"=w812, "Body"=w817, "Recipient's Email Address Address"=w816) -> ("error out"=w811:errorcluster)  [unwired: 7 in]
                  }
                }
              }
            }
            n279 = case shown="Error" w779 {
              selector: w779 -> [_ w795]
              frame No Error {
              }
              frame Error {
                w789 = " " ("string")
                n280 = Unbundle By Name(w795) -> ("code"=w792:i32)  [unwired: 2 out]
                n281 = Number To Decimal String(number=w792) -> (decimal integer string=w791:string)  [unwired: 1 in]
                n282 = Get Date/Time String() -> (date string=w794:string, time string=w793:string)  [unwired: 3 in]
                n283 = local read "Email Errors"() -> (w786:string)
                n284 = Concatenate Strings(w786, w794, w789, w793, w789, "Error" ("string"), w789, w791, "\r") -> (w787:string)
                n285 = local write "Email Errors"(w787) -> ()
              }
            }
          }
        }
      }
    }
    frame #2 {
      n286 = case shown="True" "Global Finished Email" {
        tunnel: w824 -> [_ w844]
        tunnel: w821 -> [_ w840]
        tunnel: [_ w839] -> w820
        frame False {
        }
        frame True {
          n287 = Concatenate Strings("VNA-FMR System Message " ("Subject"), w840) -> (w841:string)
          n288 = call "gmail 8.2.vi"("Subject"=w841, "Body"="All Points Finished", "Recipient's Email Address Address"=w844) -> ("error out"=w839:errorcluster)  [unwired: 8 in]
        }
      }
      n289 = call "DF Write Output String"("Write String"="F", "Communications Mode"=TRUE, "Communications On/Off"=TRUE, "GPIB Address"=w823) -> ()  [unwired: 5 in]
      n290 = local write "Status"("Finished!" ("Status")) -> ()
      n291 = case shown="Error" w820 {
        selector: w820 -> [_ w838]
        frame No Error {
        }
        frame Error {
          w832 = " " ("string")
          n292 = Unbundle By Name(w838) -> ("code"=w835:i32)  [unwired: 2 out]
          n293 = Number To Decimal String(number=w835) -> (decimal integer string=w834:string)  [unwired: 1 in]
          n294 = Get Date/Time String() -> (date string=w837:string, time string=w836:string)  [unwired: 3 in]
          n295 = local read "Email Errors"() -> (w829:string)
          n296 = Concatenate Strings(w829, w837, w832, w836, w832, "Error" ("string"), w832, w834, "\r") -> (w830:string)
          n297 = local write "Email Errors"(w830) -> ()
        }
      }
    }
    frame #3 {
      n298 = Stop(stop? (T)=TRUE) -> ()
    }
  }
  n299 = event shown="[1] \"Stop\": Value Change" {
    selector: _ -> [_ _]
    dyn-events: _ -> [_ _]
    timeout: -1 -> [_ _]
    tunnel: "Power Supply Address" -> [_ w846]
    event Timeout {
      n300 = event-data() -> ()  [unwired: 1 in, 3 out]
    }
    event "Stop": Value Change {
      n301 = event-data() -> ()  [unwired: 1 in, 6 out]
      n302 = stacked-sequence {
        tunnel: w846 -> [_ w849 _ w854 w875 _]
        frame #0 {
          n303 = Wait (ms)(milliseconds to wait=u32 250) -> ()  [unwired: 1 out]
          n304 = local write "Status"("Stopping..." ("Status")) -> ()
        }
        frame #1 {
          # "set power supply to 0 output"
          n305 = call "DF Write Output String"("Write String"="WA 00000", "Communications Mode"=TRUE, "Communications On/Off"=TRUE, "GPIB Address"=w849) -> ()  [unwired: 5 in]
        }
        frame #2 {
          n306 = Wait (ms)(milliseconds to wait=u32 100) -> ()  [unwired: 1 out]
        }
        frame #3 {
          # "Wait for\ncurrent \nto reach\nzero"
          n307 = while {
            tunnel: w854 -> [w855]
            stop <- w856 stop-if-true
            n308 = stacked-sequence {
              tunnel: [_ w866 _] -> w856
              tunnel: w855 -> [w857 w862 _]
              frame #0 {
                # "Write to power supply \"read from ch 8\""
                n309 = call "DF Write Output String"("Write String"="AD 8", "Communications Mode"=TRUE, "Communications On/Off"=TRUE, "GPIB Address"=w857) -> ()  [unwired: 5 in]
              }
              frame #1 {
                w869 = 1000.0 ("y")
                # "Read from power supply, compare to 0"
                n310 = call "DF Read Output String"("Communications Mode"=TRUE, "Readback On/Off"=TRUE, "GPIB Address"=w862) -> ("Read String"=w870:string)  [unwired: 4 in, 1 out]
                n311 = Decimal String To Number(string=w870, offset=1, default (0L)=w869) -> (number=w868:dbl)  [unwired: 1 out]
                n312 = Divide(x=w868, y=w869) -> (x/y=w864:dbl)
                n313 = Subtract(x=w864, y=0.001) -> (x-y=w863:dbl)
                n314 = Less Or Equal?(x=w863, y=0.0) -> (x <= y?=w866:bool)
              }
              frame #2 {
                n315 = Wait (ms)(milliseconds to wait=u32 100) -> ()  [unwired: 1 out]
              }
            }
          }
        }
        frame #4 {
          # "Turn off power supply"
          n316 = local write "Status"("Stopped." ("Status")) -> ()
          n317 = call "DF Write Output String"("Write String"="F", "Communications Mode"=TRUE, "Communications On/Off"=TRUE, "GPIB Address"=w875) -> ()  [unwired: 5 in]
        }
        frame #5 {
          # "end program"
          n318 = Stop(stop? (T)=TRUE) -> ()
        }
      }
    }
  }
